vi "一体站流程自动启动.vi"(11 "参数":T1={"CODCr"={"启动测量模式"={"测量模式"=enum."水样测量"}, "确定按钮"=TRUE}, "参数启用"={"多参数"=FALSE, "CODMn"=FALSE, "总磷总氮"=FALSE, "氨氮"=FALSE, "CODcr"=FALSE}}) -> ()   [LabVIEW 2016, in "PLC.lvlib"]
uses:
  PLC.lvlib
  API/CodCr/CodCr.lvlib
panel:
  out "枚举":enum16{"初始化", "采配水启动", "等待", "配水", "排水", "结束"}(ring)
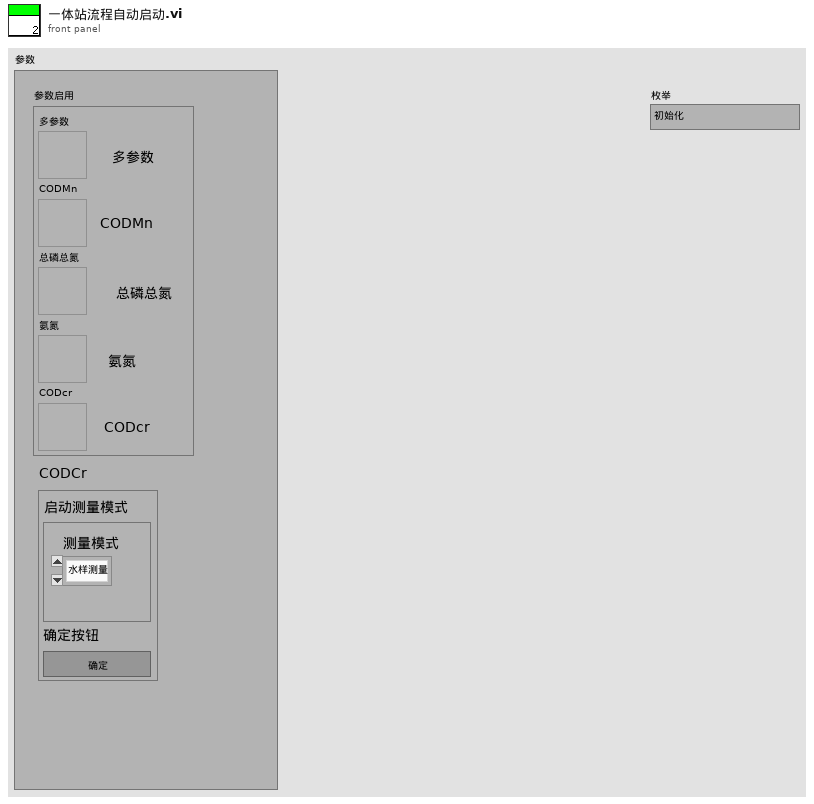
[diagram p1: front panel]
types:
  T1 = cluster{"CODCr":cluster{"启动测量模式":cluster{"测量模式":enum16{"水样测量", "标样核查", "零点核查", "跨度核查", "空白测试", "加标回收", "平行样", "校零", "校标"}}, "确定按钮":bool}, "参数启用":cluster{"多参数":bool, "CODMn":bool, "总磷总氮":bool, "氨氮":bool, "CODcr":bool}}
  T2 = cluster{"命令":string, cluster{"starting address":u16, "holding register value":u16}}
  T3 = cluster{"测量模式":enum16{"水样测量", "标样核查", "零点核查", "跨度核查", "空白测试", "加标回收", "平行样", "校零", "校标"}}
  T4 = cluster{"时间标识":timestamp, "设备":string, "日志信息":string, "流程参数":string}
  T5 = cluster{"时间标识":timestamp, "设备":string, "日志信息":string}
  T6 = enum16{"空闲", "水样测试", "标样核查", "零点核查", "跨度核查", "空白测试", "平行样测试", "加标回收", "空白校准", "标样校准", "初始化（清洗）"}
  T7 = enum16{"待机", "启动氨氮", "氨氮测量中", "启动总磷", "总磷测量中", "结束"}
  T8 = cluster{"站号":u16, "量程切换":enum32{"H", "L", "AUTO"}, "控制命令":enum16{"启动测量", "标样核查", "零点核查", "跨度核查", "空白测试", "平行样测试", "加标回收", "空白校准", "标样校准", "初始化（清洗）", "停止测试", "仪器重启", "校时", "模式设置", "测量间隔设置"}, "模式设置":enum16{"待机", "连续模式", "周期模式", "定点模式", "受控模式", "手动模式"}, "测量间隔":u16}
  T9 = cluster{"测量模式":enum16{"待机", "水样测试", "标样核查", "零点核查", "跨度核查", "空白测试", "平行样测试", "加标回收", "空白校准", "标样校准", "初始化（清洗）"}, "数据标记表":string, "测量时间":dbl}
  T10 = enum16{"待机", "水样测试", "标样核查", "零点核查", "跨度核查", "空白测试", "平行样测试", "加标回收", "空白校准", "标样校准", "初始化（清洗）"}
  T11 = cluster{"R0":i16, "R1":i16, "R2":i16, "R3":i16, "R4":i16, "R5":i16, "R6":i16, "R7":i16, "R8":i16, "R9":i16, "R10":i16, "R11":i16, "R12":i16, "R13":i16, "R14":i16, "R15":i16, "R16":i16, "R17":i16, "R18":i16, "R19":i16, "R20":i16, "R21":i16, "R22":i16, "R23":i16, "R24":i16, "R25":i16, "R26":i16, "R27":i16, "R28":i16, "R29":i16, "R30":i16, "R31":i16, "R32":i16, "R33":i16, "R34":i16, "R35":i16, "R36":i16, "R37":i16, "R38":i16, "R39":i16, "R40":i16, "R41":i16, "R42":i16, "R43":i16, "R44":i16, "R45":i16, "R46":i16, "R47":i16, "R48":i16, "R49":i16, "R50":i16, "R51":i16, "R52":i16, "R53":i16, "R54":i16, "R55":i16}
  T12 = cluster{"系统时间":timestamp, "工作状态":enum16{"空闲", "水样测试", "标样核查", "零点核查", "跨度核查", "空白测试", "平行样测试", "加标回收", "空白校准", "标样校准", "初始化（清洗）"}, "测量模式":enum16{"待机", "连续模式", "周期模式", "定点模式", "受控模式", "手动模式"}, "告警代码":enum16{"无告警", "缺试剂告警", "缺水样告警", "缺蒸馏水告警", "缺标液告警", "仪表漏液告警", "标定异常告警", "超量程告警", "加热异常", "低试剂预警", "超上限告警", "超下限告警", "仪表内部其他异常", "滴定异常告警", "电极异常告警", "量程切换告警", "参数设置告警", "PH电极电位异常", "电导率电极异常", "浊度光度异常", "溶解氧电极异常", "溶解氧光强异常", "温度异常告警", "PH异常告警", "溶解氧异常告警", "电导率异常告警", "浊度异常告警", "叶绿素异常告警", "藻密度异常告警", "蓝绿藻异常告警", "ORP异常告警", "氨氮异常告警", "清洁刷异常告警", "SD卡异常告警", "蓝牙异常告警", "Wifi异常告警", "流程异常告警"}, "故障代码":enum16{"无故障", "电机故障", "温度故障", "通讯故障", "滴定故障"}, "日志代码":u16, "软件版本":u16, "F0":sgl, "F1":sgl, "F2":sgl, "F3":sgl, "T":sgl, "H":sgl, "id":u16, "flowid":u16, "量程":u16, "总磷控温温度1":sgl, "营养盐控温温度2":sgl, "ADC":sgl}
  T13 = cluster{"因子编码":u32, "单位":u16, "标样参考值":sgl, "水样数据时间":timestamp, "水样实测值":sgl, "水样数据标识":string, "标样数据时间":timestamp, "标样实测值":sgl, "标样数据标识":string, "空白数据时间":timestamp, "空白实测值":sgl, "空白数据标识":string, "零点核查数据时间":timestamp, "零点核查实测值":sgl, "零点核查数据标识":string, "跨度核查数据时间":timestamp, "跨度核查实测值":sgl, "跨度核查数据标识":string, "加标回收数据时间":timestamp, "加标回收实测值":sgl, "加标回收数据标识":string, "平行样数据时间":timestamp, "平行样实测值":sgl, "平行样数据标识":string, "F0":sgl, "F1":sgl, "F2":sgl, "F3":sgl, "F4":sgl, "F5":sgl, "F6":sgl, "F7":sgl, "温度":sgl, "湿度":sgl, "X值":sgl}
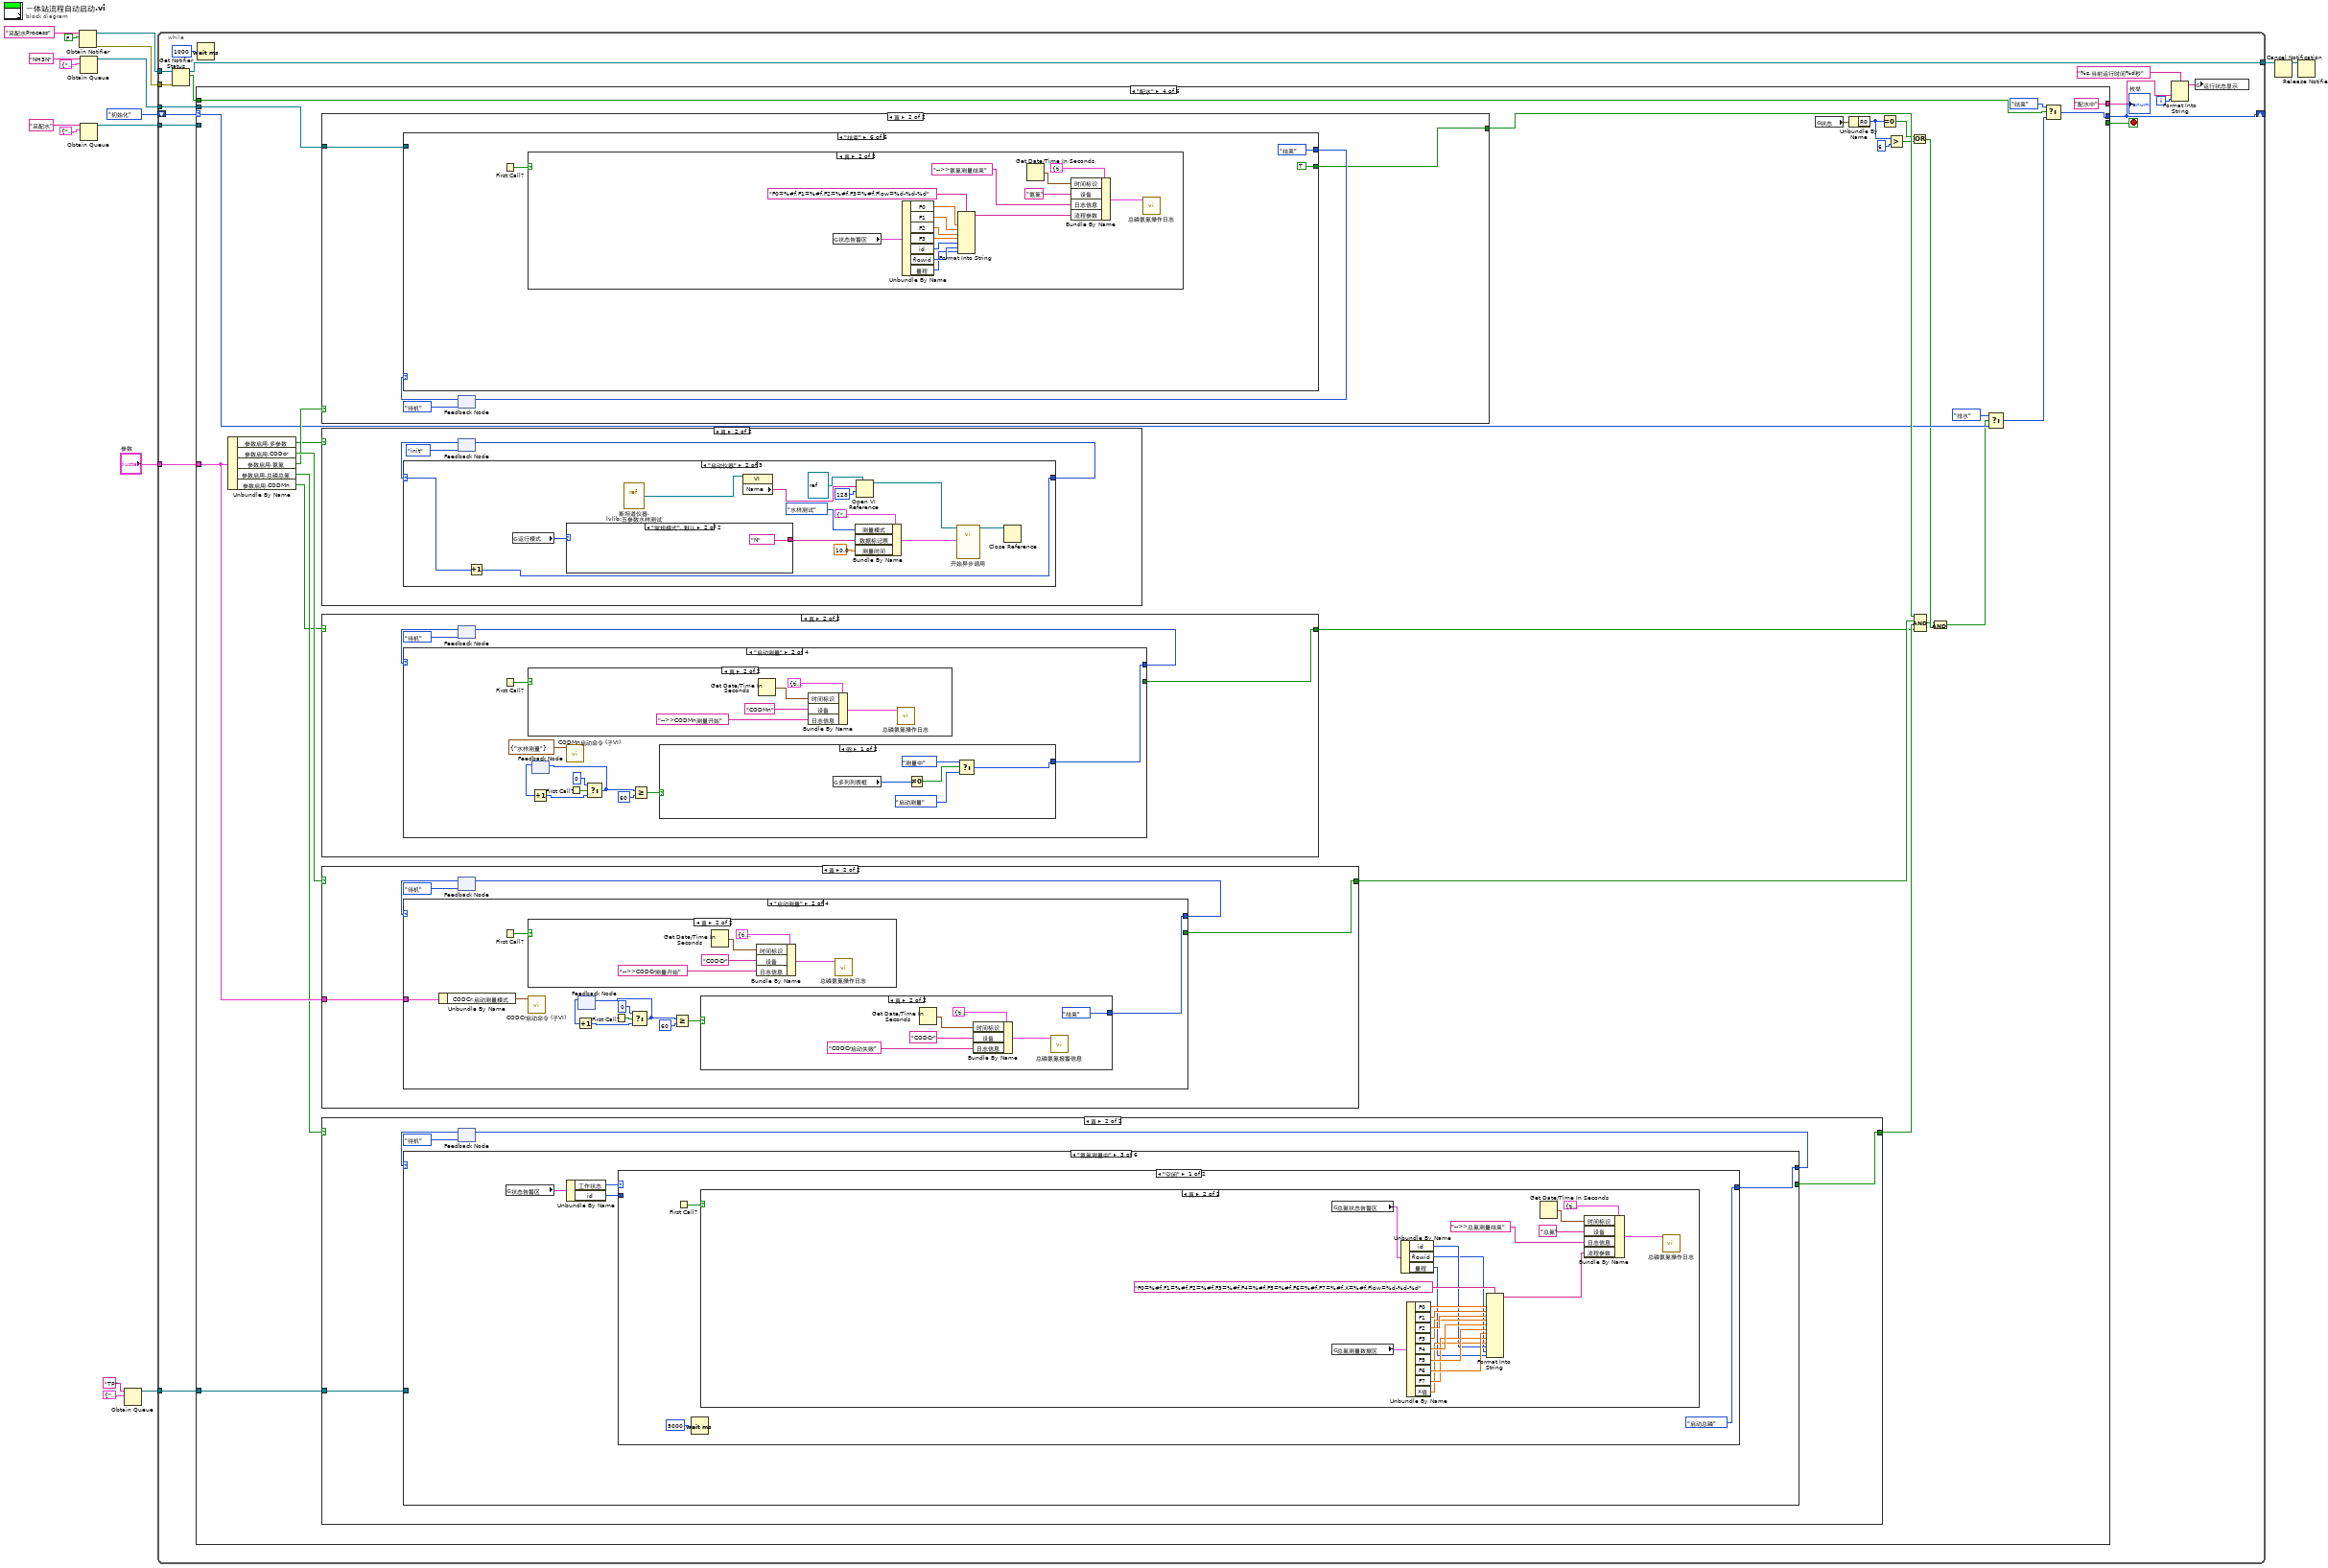
[diagram p0: block diagram]
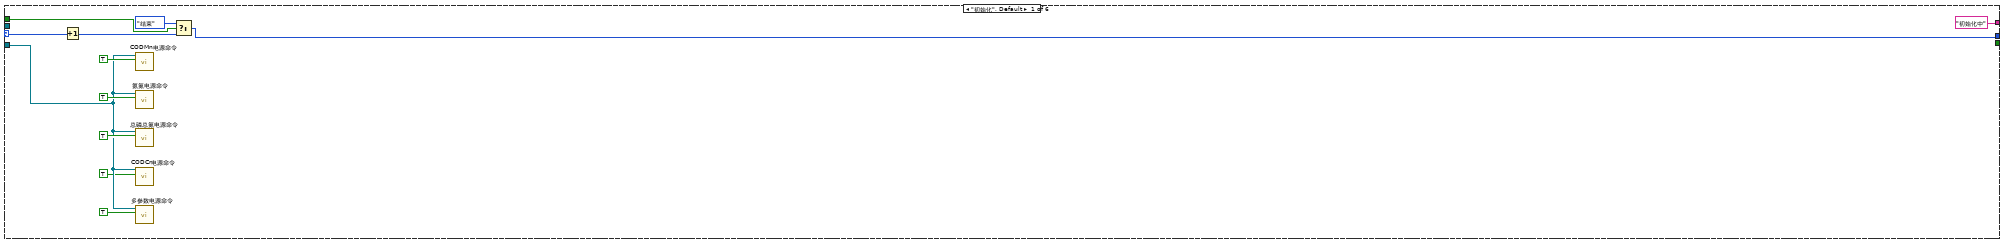
[diagram p2: hidden frame]
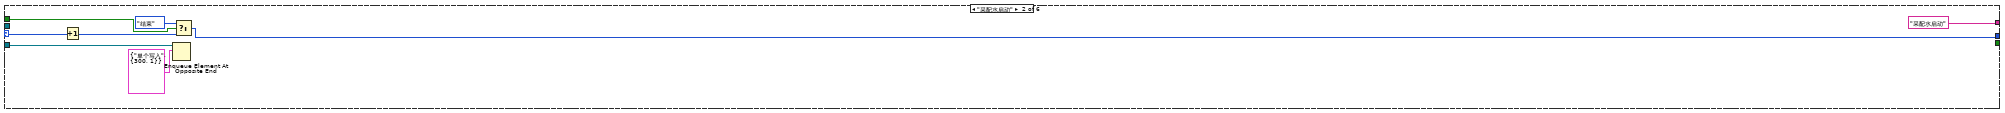
[diagram p3: hidden frame]
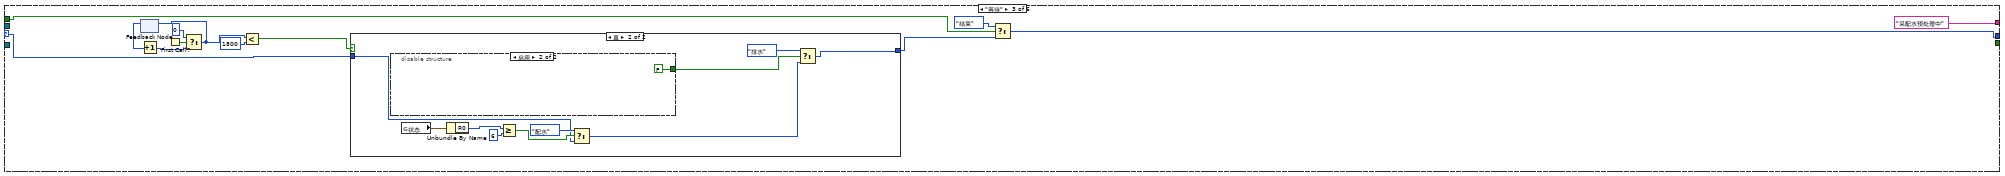
[diagram p4: hidden frame]
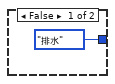
[diagram p5: hidden frame]
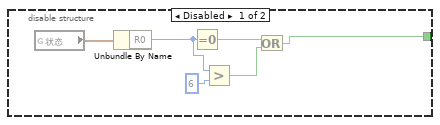
[diagram p6: hidden frame]
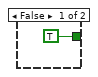
[diagram p7: hidden frame]
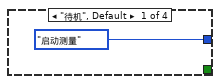
[diagram p8: hidden frame]
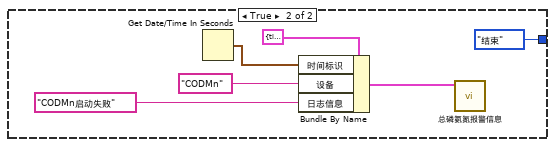
[diagram p10: hidden frame]
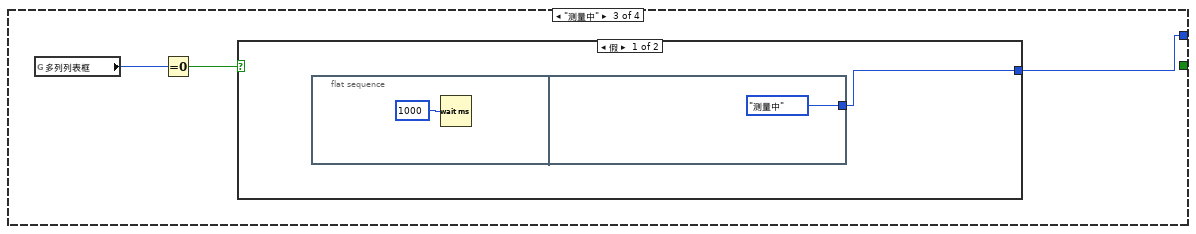
[diagram p11: hidden frame]
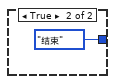
[diagram p12: hidden frame]
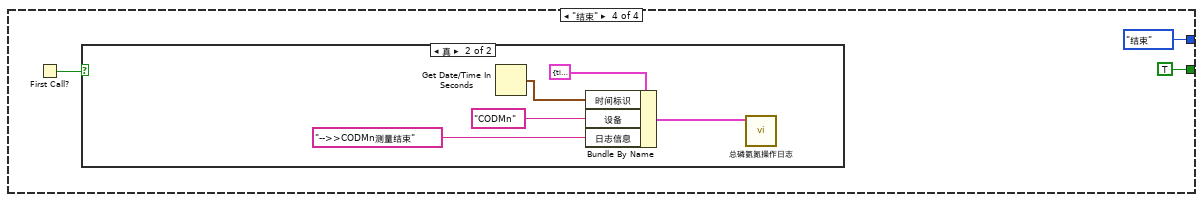
[diagram p13: hidden frame]
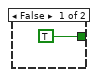
[diagram p15: hidden frame]
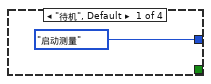
[diagram p16: hidden frame]
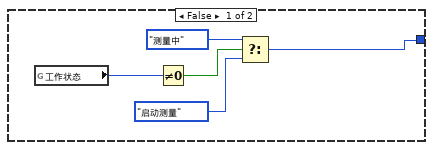
[diagram p18: hidden frame]
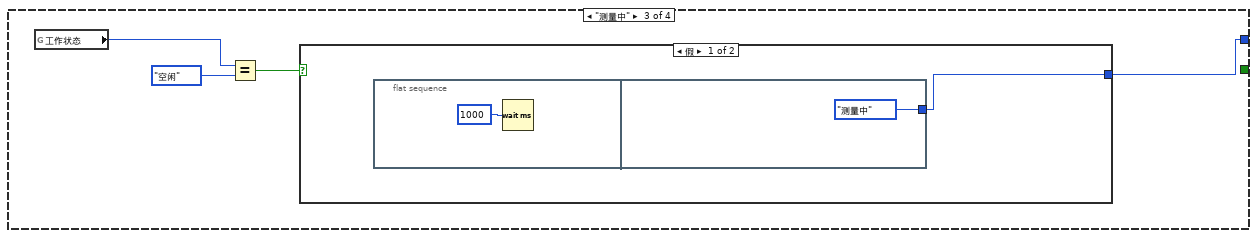
[diagram p19: hidden frame]
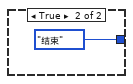
[diagram p20: hidden frame]
diagram:
  n1 = Obtain Notifier(name (unnamed)="采配水Process" ("名称（未命名）"), notification data type=FALSE) -> (notifier out=w2:refnum<notifier>, error out=w1:errorcluster)  [unwired: 2 in, 1 out]
  n2 = Obtain Queue(name (unnamed)="NH3N" ("名称（未命名）"), element data type=cluster{"命令":string, "data":variant} {"命令"="", "data"=variant}) -> (queue out=w4:refnum<queue>)  [unwired: 3 in, 2 out]
  n3 = Obtain Queue(name (unnamed)="采配水" ("名称（未命名）"), element data type=cluster{"命令":string, "数据":variant} {"命令"="", "数据"=variant}) -> (queue out=w15:refnum<queue>)  [unwired: 3 in, 2 out]
  n4 = Obtain Queue(name (unnamed)="TP" ("名称（未命名）"), element data type=cluster{"命令":string, "data":variant} {"命令"="", "data"=variant}) -> (queue out=w3:refnum<queue>)  [unwired: 3 in, 2 out]
  n5 = while {
    tunnel: w15 -> [w33]
    shift-right: [w31] -> _
    shift-left: enum16{"初始化", "采配水启动", "等待", "配水", "排水", "结束"}."初始化" ("枚举") -> [w32]
    tunnel: w4 -> [w29]
    tunnel: "参数" -> [w28]
    tunnel: w2 -> [w27]
    tunnel: [w26] -> w8
    tunnel: w3 -> [w21]
    tunnel: w1 -> [w18]
    i -> [w23]
    stop <- w19 stop-if-true
    n6 = Get Notifier Status(notifier=w27, error in (no error)=w18) -> (notifier out=w26:refnum<notifier>, current notification=w22:bool)  [unwired: 3 out]
    n7 = case shown="\"配水\"" w32 {
      selector: w32 -> [w45 w51 w64 w89 w497 w505]
      tunnel: w33 -> [w35 w52 _ _ w498 w501]
      tunnel: [w41 w46 w54 w108 w492 w504] -> w31
      tunnel: [_ _ _ _ _ TRUE] -> w19
      tunnel: w29 -> [_ _ _ w106 _ _]
      tunnel: w28 -> [_ _ _ w103 _ _]
      tunnel: ["初始化中" ("输入 1") "采配水启动" ("输入 1") "采配水预处理中" ("输入 1") "配水中" ("输入 1") "排水中" ("输入 1") "结束" ("输入 1")] -> w24
      tunnel: w22 -> [w43 w48 w56 w109 w494 w500]
      tunnel: w21 -> [_ _ _ w107 _ _]
      frame "初始化", Default {
        n8 = Increment(x=w45) -> (x+1=w42:enum16{"初始化", "采配水启动", "等待", "配水", "排水", "结束"})
        n9 = call "CODMn电源命令.vi"("通电/断电"=TRUE, "队列"=w35) -> ()  [unwired: 9 in, 1 out]
        n10 = call "氨氮电源命令.vi"("通电/断电"=TRUE, "队列"=w35) -> ()  [unwired: 9 in, 1 out]
        n11 = call "总磷总氮电源命令.vi"("通电/断电"=TRUE, "队列"=w35) -> ()  [unwired: 9 in, 1 out]
        n12 = call "CODCr电源命令.vi"("通电/断电"=TRUE, "队列"=w35) -> ()  [unwired: 9 in, 1 out]
        n13 = call "多参数电源命令.vi"("通电/断电"=TRUE, "队列"=w35) -> ()  [unwired: 9 in, 1 out]
        n14 = Select(t=enum16{"初始化", "采配水启动", "等待", "配水", "排水", "结束"}."结束", s=w43, f=w42) -> (s? t:f=w41:enum16{"初始化", "采配水启动", "等待", "配水", "排水", "结束"})
      }
      frame "采配水启动" {
        n15 = Increment(x=w51) -> (x+1=w47:enum16{"初始化", "采配水启动", "等待", "配水", "排水", "结束"})
        n16 = Enqueue Element At Opposite End(queue=w52, element=T2 {"命令"="单个写入", {"starting address"=300, "holding register value"=1}} ("元素")) -> ()  [unwired: 2 in, 3 out]
        n17 = Select(t=enum16{"初始化", "采配水启动", "等待", "配水", "排水", "结束"}."结束", s=w48, f=w47) -> (s? t:f=w46:enum16{"初始化", "采配水启动", "等待", "配水", "排水", "结束"})
      }
      frame "等待" {
        n18 = feedback #1() -> (w61:i32)  [unwired: 1 in]
        n19 = Increment(x=w61) -> (x+1=w60:i32)
        n20 = First Call?() -> (First Call?: T/F=w62:bool)
        n21 = Select(t=0, s=w62, f=w60) -> (s? t:f=w59:i32)
        n22 = feedback-in #1(w59) -> ()
        n23 = Less?(x=w59, y=1800) -> (x < y?=w65:bool)
        n24 = case shown="真" w65 {
          tunnel: w64 -> [_ w70]
          tunnel: [enum16{"初始化", "采配水启动", "等待", "配水", "排水", "结束"}."排水" ("枚举") w68] -> w55
          frame False {
          }
          frame True {
            n25 = disable-structure shown="启用" {
              disable-tunnel: [w83 FALSE] -> w72
              frame Disabled {
                n26 = global read "采配水全局变量.vi" "状态"() -> (w78:T11)
                n27 = Unbundle By Name(w78) -> ("R0"=w79:i16)
                n28 = Equal To 0?(x=w79) -> (x = 0?=w82:bool)
                n29 = Greater?(x=w79, y=i16 6) -> (0:w81:bool)
                n30 = Or(x=w82, y=w81) -> (x .or. y?=w83:bool)
              }
              frame Enabled {
              }
            }
            n31 = global read "采配水全局变量.vi" "状态"() -> (w77:T11)
            n32 = Unbundle By Name(w77) -> ("R0"=w76:i16)
            n33 = Greater Or Equal?(x=w76, y=i16 6) -> (x >= y?=w74:bool)
            n34 = Select(t=enum16{"初始化", "采配水启动", "等待", "配水", "排水", "结束"}."配水" ("枚举"), s=w74, f=w70) -> (s? t:f=w69:enum16{"初始化", "采配水启动", "等待", "配水", "排水", "结束"})
            n35 = Select(t=enum16{"初始化", "采配水启动", "等待", "配水", "排水", "结束"}."排水" ("枚举"), s=w72, f=w69) -> (s? t:f=w68:enum16{"初始化", "采配水启动", "等待", "配水", "排水", "结束"})
          }
        }
        n36 = Select(t=enum16{"初始化", "采配水启动", "等待", "配水", "排水", "结束"}."结束", s=w56, f=w55) -> (s? t:f=w54:enum16{"初始化", "采配水启动", "等待", "配水", "排水", "结束"})
      }
      frame "配水" {
        n37 = Unbundle By Name(w103) -> ("参数启用.多参数"=w96:bool, "参数启用.CODcr"=w100:bool, "参数启用.氨氮"=w99:bool, "参数启用.总磷总氮"=w98:bool, "参数启用.CODMn"=w97:bool)
        n38 = case shown="真" w99 {
          tunnel: [TRUE w367] -> w105
          tunnel: w106 -> [_ w366]
          frame False {
          }
          frame True {
            n39 = feedback #2(T7."待机") -> (w369:T7)
            n40 = case shown="\"结束\"" w369 {
              tunnel: [T7."启动氨氮" w383 w412 w430 w444 T7."结束"] -> w368
              tunnel: [_ _ _ _ _ TRUE] -> w367
              tunnel: w366 -> [_ w374 _ w421 _ _]
              frame "待机", Default {
              }
              frame "启动氨氮" {
                n41 = First Call?() -> (First Call?: T/F=w372:bool)
                n42 = case shown="真" w372 {
                  frame False {
                  }
                  frame True {
                    n43 = global read "VAR总磷氨氮全局变量.vi" "状态告警区"() -> (w393:T12)
                    n44 = Unbundle By Name(w393) -> ("F0"=w391:sgl, "F1"=w390:sgl, "F2"=w389:sgl, "F3"=w388:sgl, "id"=w387:u16, "flowid"=w386:u16, "量程"=w385:u16)
                    n45 = Format Into String(format string="F0=%#f,F1=%#f,F2=%#f,F3=%#f,%d-%d-%d" ("格式字符串"), w391, w390, w389, w388, w387, w386, w385) -> (resulting string=w384:string)  [unwired: 2 in, 1 out]
                    n46 = Get Date/Time In Seconds() -> (seconds since 1Jan1904=w396:timestamp)
                    n47 = Bundle By Name(cluster=T4 {"时间标识"=timestamp(0 s since 1904-01-01), "设备"="", "日志信息"="", "流程参数"=""} ("data in"), "时间标识"=w396, "设备"="氨氮", "日志信息"="-->>氨氮测量开始" ("设备"), "流程参数"=w384) -> (w397:T4)
                    n48 = call "总磷氨氮操作日志.vi"("data in"=w397) -> ()  [unwired: 11 in]
                  }
                }
                n49 = call "总磷氨氮启动命令.vi"("参数"=T8 {"站号"=3, "量程切换"=enum."AUTO", "控制命令"=enum."启动测量", "模式设置"=enum."待机", "测量间隔"=0}) -> ("启动命令"=w375:cluster{"命令":string, "data":variant})  [unwired: 10 in]
                n50 = Enqueue Element(queue=w374, element=w375) -> ()  [unwired: 2 in, 3 out]
                n51 = feedback #3() -> (w380:i32)  [unwired: 1 in]
                n52 = Increment(x=w380) -> (x+1=w379:i32)
                n53 = First Call?() -> (First Call?: T/F=w381:bool)
                n54 = Select(t=0, s=w381, f=w379) -> (s? t:f=w378:i32)
                n55 = feedback-in #3(w378) -> ()
                n56 = Greater Or Equal?(x=w378, y=60) -> (x >= y?=w376:bool)
                n57 = case shown="真" w376 {
                  tunnel: [w402 T7."结束"] -> w383
                  frame False {
                    n58 = global read "VAR总磷氨氮全局变量.vi" "状态告警区"() -> (w399:T12)
                    n59 = Unbundle By Name(w399) -> ("工作状态"=w404:T6)
                    n60 = Not Equal To 0?(x=w404) -> (x != 0?=w403:bool)
                    n61 = Select(t=T7."氨氮测量中", s=w403, f=T7."启动氨氮") -> (s? t:f=w402:T7)
                  }
                  frame True {
                    n62 = Get Date/Time In Seconds() -> (seconds since 1Jan1904=w409:timestamp)
                    n63 = Bundle By Name(cluster=T5 {"时间标识"=timestamp(0 s since 1904-01-01), "设备"="", "日志信息"=""} ("data in"), "时间标识"=w409, "设备"="氨氮", "日志信息"="氨氮启动失败") -> (w405:T5)
                    n64 = call "总磷氨氮报警信息.vi"("data in"=w405) -> ()  [unwired: 11 in]
                  }
                }
              }
              frame "氨氮测量中" {
                n65 = global read "VAR总磷氨氮全局变量.vi" "状态告警区"() -> (w411:T12)
                n66 = Unbundle By Name(w411) -> ("工作状态"=w414:T6, "id"=w413:u16)
                n67 = case shown="\"水样测试\", 默认" w414 {
                  tunnel: [T7."结束" w416] -> w412
                  tunnel: w413 -> [_ w417]
                  frame "空闲" {
                  }
                  frame "水样测试", Default {
                    n68 = case shown="76, 默认" w417 {
                      tunnel: [T7."氨氮测量中" T7."总磷测量中"] -> w416
                      frame 76, Default {
                      }
                      frame 131 {
                      }
                    }
                  }
                }
              }
              frame "启动总磷" {
                n69 = call "总磷氨氮启动命令.vi"("参数"=T8 {"站号"=1, "量程切换"=enum."AUTO", "控制命令"=enum."启动测量", "模式设置"=enum."待机", "测量间隔"=0}) -> ("启动命令"=w422:cluster{"命令":string, "data":variant})  [unwired: 10 in]
                n70 = Enqueue Element(queue=w421, element=w422) -> ()  [unwired: 2 in, 3 out]
                n71 = feedback #4() -> (w427:i32)  [unwired: 1 in]
                n72 = Increment(x=w427) -> (x+1=w426:i32)
                n73 = First Call?() -> (First Call?: T/F=w428:bool)
                n74 = Select(t=0, s=w428, f=w426) -> (s? t:f=w425:i32)
                n75 = feedback-in #4(w425) -> ()
                n76 = Greater Or Equal?(x=w425, y=60) -> (x >= y?=w423:bool)
                n77 = case shown="假" w423 {
                  tunnel: [w434 T7."结束"] -> w430
                  frame False {
                    n78 = global read "VAR总磷氨氮全局变量.vi" "状态告警区"() -> (w431:T12)
                    n79 = Unbundle By Name(w431) -> ("工作状态"=w435:T6)
                    n80 = Not Equal To 0?(x=w435) -> (x != 0?=w436:bool)
                    n81 = Select(t=T7."总磷测量中", s=w436, f=T7."启动总磷") -> (s? t:f=w434:T7)
                  }
                  frame True {
                    n82 = Get Date/Time In Seconds() -> (seconds since 1Jan1904=w442:timestamp)
                    n83 = Bundle By Name(cluster=T5 {"时间标识"=timestamp(0 s since 1904-01-01), "设备"="", "日志信息"=""} ("data in"), "时间标识"=w442, "设备"="总磷", "日志信息"="总磷启动失败") -> (w437:T5)
                    n84 = call "总磷氨氮报警信息.vi"("data in"=w437) -> ()  [unwired: 11 in]
                  }
                }
              }
              frame "总磷测量中" {
                n85 = global read "VAR总磷氨氮全局变量.vi" "状态告警区"() -> (w443:T12)
                n86 = Unbundle By Name(w443) -> ("工作状态"=w446:T6, "id"=w445:u16)
                n87 = case shown="\"水样测试\", 默认" w446 {
                  tunnel: [T7."结束" w448] -> w444
                  tunnel: w445 -> [_ w449]
                  frame "空闲" {
                  }
                  frame "水样测试", Default {
                    n88 = case shown="76, 默认" w449 {
                      tunnel: [T7."氨氮测量中" T7."总磷测量中"] -> w448
                      frame 76, Default {
                      }
                      frame 131 {
                      }
                    }
                  }
                }
              }
              frame "结束" {
                n89 = First Call?() -> (First Call?: T/F=w452:bool)
                n90 = case shown="真" w452 {
                  frame False {
                  }
                  frame True {
                    n91 = global read "VAR总磷氨氮全局变量.vi" "状态告警区"() -> (w464:T12)
                    n92 = Unbundle By Name(w464) -> ("F0"=w462:sgl, "F1"=w461:sgl, "F2"=w460:sgl, "F3"=w459:sgl, "id"=w458:u16, "flowid"=w457:u16, "量程"=w456:u16)
                    n93 = Format Into String(format string="F0=%#f,F1=%#f,F2=%#f,F3=%#f,Flow=%d-%d-%d" ("格式字符串"), w462, w461, w460, w459, w458, w457, w456) -> (resulting string=w455:string)  [unwired: 2 in, 1 out]
                    n94 = Get Date/Time In Seconds() -> (seconds since 1Jan1904=w467:timestamp)
                    n95 = Bundle By Name(cluster=T4 {"时间标识"=timestamp(0 s since 1904-01-01), "设备"="", "日志信息"="", "流程参数"=""} ("data in"), "时间标识"=w467, "设备"="氨氮", "日志信息"="-->>氨氮测量结束" ("设备"), "流程参数"=w455) -> (w468:T4)
                    n96 = call "总磷氨氮操作日志.vi"("data in"=w468) -> ()  [unwired: 11 in]
                  }
                }
              }
            }
            n97 = feedback-in #2(w368) -> ()
          }
        }
        n98 = case shown="真" w96 {
          frame False {
          }
          frame True {
            n99 = feedback #5(enum16{"init", "启动仪器", "测量中"}."init") -> (w471:enum16{"init", "启动仪器", "测量中"})
            n100 = case shown="\"启动仪器\"" w471 {
              selector: w471 -> [w474 w488 _]
              tunnel: [w473 w487 enum16{"init", "启动仪器", "测量中"}."测量中"] -> w472
              frame "init", Default {
                n101 = Increment(x=w474) -> (x+1=w473:enum16{"init", "启动仪器", "测量中"})
              }
              frame "启动仪器" {
                n102 = Increment(x=w488) -> (x+1=w487:enum16{"init", "启动仪器", "测量中"})
                n103 = global read "系统变量.vi" "运行模式"() -> (w476:enum16{"维护模式", "常规模式", "应急模式", "质控模式"})
                n104 = case shown="\"常规模式\", 默认" w476 {
                  tunnel: ["M" ("数据标记表") "N" ("数据标记表")] -> w475
                  frame "维护模式" {
                  }
                  frame "常规模式", Default {
                  }
                }
                n105 = vi-ref "斯坦道仪器.lvlib:五参数水样测试.vi"() -> (w486:refnum<vi>)
                n106 = property class="VI"(reference=w486) -> ("Name"=w485:string)  [unwired: 1 in, 2 out]
                n107 = Bundle By Name(cluster=T9 {"测量模式"=enum."待机", "数据标记表"="", "测量时间"=0.0} ("启动参数"), "测量模式"=T10."水样测试", "数据标记表"=w475, "测量时间"=10.0) -> (w477:T9)
                n108 = Open VI Reference(type specifier VI Refnum (for type only)=refnum<vi> refnum ("类型说明符VI引用句柄（仅用于类型）"), vi path=w485, options=128 ("选项")) -> (vi reference=w480:refnum<vi>)  [unwired: 3 in, 1 out]
                n109 = call-by-ref "开始异步调用"(reference=w480, "启动参数"=w477) -> (reference out=w479:refnum<vi>)  [unwired: 12 in, 1 out]
                n110 = Close Reference(reference=w479) -> ()  [unwired: 1 in, 1 out]
              }
              frame "测量中" {
              }
            }
            n111 = feedback-in #5(w472) -> ()
          }
        }
        n112 = case shown="真" w97 {
          tunnel: [TRUE w113] -> w101
          frame False {
          }
          frame True {
            n113 = feedback #6(enum16{"待机", "启动测量", "测量中", "结束"}."待机") -> (w115:enum16{"待机", "启动测量", "测量中", "结束"})
            n114 = case shown="\"启动测量\"" w115 {
              tunnel: [enum16{"待机", "启动测量", "测量中", "结束"}."启动测量" w127 w146 enum16{"待机", "启动测量", "测量中", "结束"}."结束"] -> w114
              tunnel: [_ _ _ TRUE] -> w113
              frame "待机", Default {
              }
              frame "启动测量" {
                n115 = First Call?() -> (First Call?: T/F=w118:bool)
                n116 = case shown="真" w118 {
                  frame False {
                  }
                  frame True {
                    n117 = Get Date/Time In Seconds() -> (seconds since 1Jan1904=w132:timestamp)
                    n118 = Bundle By Name(cluster=T4 {"时间标识"=timestamp(0 s since 1904-01-01), "设备"="", "日志信息"="", "流程参数"=""} ("data in"), "时间标识"=w132, "设备"="CODMn", "日志信息"="-->>CODMn测量开始") -> (w128:T4)
                    n119 = call "总磷氨氮操作日志.vi"("data in"=w128) -> ()  [unwired: 11 in]
                  }
                }
                n120 = feedback #7() -> (w123:i32)  [unwired: 1 in]
                n121 = Increment(x=w123) -> (x+1=w124:i32)
                n122 = call "CODMn启动命令 (子VI).vi"("启动测量模式"=T3 {"测量模式"=enum."水样测量"}) -> ()  [unwired: 11 in]
                n123 = First Call?() -> (First Call?: T/F=w122:bool)
                n124 = Select(t=0, s=w122, f=w124) -> (s? t:f=w125:i32)
                n125 = feedback-in #7(w125) -> ()
                n126 = Greater Or Equal?(x=w125, y=60) -> (x >= y?=w120:bool)
                n127 = case shown="假" w120 {
                  tunnel: [w134 enum16{"待机", "启动测量", "测量中", "结束"}."结束"] -> w127
                  frame False {
                    n128 = global read "运行时序全局变量.vi" "多列列表框"() -> (w133:i32)
                    n129 = Not Equal To 0?(x=w133) -> (x != 0?=w135:bool)
                    n130 = Select(t=enum16{"待机", "启动测量", "测量中", "结束"}."测量中", s=w135, f=enum16{"待机", "启动测量", "测量中", "结束"}."启动测量") -> (s? t:f=w134:enum16{"待机", "启动测量", "测量中", "结束"})
                  }
                  frame True {
                    n131 = Get Date/Time In Seconds() -> (seconds since 1Jan1904=w138:timestamp)
                    n132 = Bundle By Name(cluster=T5 {"时间标识"=timestamp(0 s since 1904-01-01), "设备"="", "日志信息"=""} ("data in"), "时间标识"=w138, "设备"="CODMn", "日志信息"="CODMn启动失败") -> (w142:T5)
                    n133 = call "总磷氨氮报警信息.vi"("data in"=w142) -> ()  [unwired: 11 in]
                  }
                }
              }
              frame "测量中" {
                n134 = global read "运行时序全局变量.vi" "多列列表框"() -> (w145:i32)
                n135 = Equal To 0?(x=w145) -> (x = 0?=w144:bool)
                n136 = case shown="假" w144 {
                  tunnel: [w147 enum16{"待机", "启动测量", "测量中", "结束"}."结束"] -> w146
                  frame False {
                    n137 = flat-sequence {
                      tunnel: [enum16{"待机", "启动测量", "测量中", "结束"}."测量中"] -> w147
                      frame #0 {
                        n138 = Wait (ms)(milliseconds to wait=u32 1000 ("等待时间（毫秒）")) -> ()  [unwired: 1 out]
                      }
                      frame #1 {
                      }
                    }
                  }
                  frame True {
                  }
                }
              }
              frame "结束" {
                n139 = First Call?() -> (First Call?: T/F=w151:bool)
                n140 = case shown="真" w151 {
                  frame False {
                  }
                  frame True {
                    n141 = Get Date/Time In Seconds() -> (seconds since 1Jan1904=w158:timestamp)
                    n142 = Bundle By Name(cluster=T4 {"时间标识"=timestamp(0 s since 1904-01-01), "设备"="", "日志信息"="", "流程参数"=""} ("data in"), "时间标识"=w158, "设备"="CODMn", "日志信息"="-->>CODMn测量结束") -> (w154:T4)
                    n143 = call "总磷氨氮操作日志.vi"("data in"=w154) -> ()  [unwired: 11 in]
                  }
                }
              }
            }
            n144 = feedback-in #6(w114) -> ()
          }
        }
        n145 = case shown="真" w100 {
          tunnel: [TRUE w161] -> w102
          tunnel: w103 -> [_ w160]
          frame False {
          }
          frame True {
            n146 = feedback #8(enum16{"待机", "启动测量", "测量中", "结束"}."待机") -> (w163:enum16{"待机", "启动测量", "测量中", "结束"})
            n147 = case shown="\"启动测量\"" w163 {
              tunnel: [enum16{"待机", "启动测量", "测量中", "结束"}."启动测量" w175 w196 enum16{"待机", "启动测量", "测量中", "结束"}."结束"] -> w162
              tunnel: w160 -> [_ w176 _ _]
              tunnel: [_ _ _ TRUE] -> w161
              frame "待机", Default {
              }
              frame "启动测量" {
                n148 = Unbundle By Name(w176) -> ("CODCr.启动测量模式"=w174:T3)
                n149 = First Call?() -> (First Call?: T/F=w166:bool)
                n150 = case shown="真" w166 {
                  frame False {
                  }
                  frame True {
                    n151 = Get Date/Time In Seconds() -> (seconds since 1Jan1904=w181:timestamp)
                    n152 = Bundle By Name(cluster=T4 {"时间标识"=timestamp(0 s since 1904-01-01), "设备"="", "日志信息"="", "流程参数"=""} ("data in"), "时间标识"=w181, "设备"="CODCr", "日志信息"="-->>CODCr测量开始") -> (w177:T4)
                    n153 = call "总磷氨氮操作日志.vi"("data in"=w177) -> ()  [unwired: 11 in]
                  }
                }
                n154 = call "CODCr启动命令 (子VI).vi"("启动测量模式"=w174) -> ()  [unwired: 11 in]
                n155 = feedback #9() -> (w170:i32)  [unwired: 1 in]
                n156 = Increment(x=w170) -> (x+1=w171:i32)
                n157 = First Call?() -> (First Call?: T/F=w169:bool)
                n158 = Select(t=0, s=w169, f=w171) -> (s? t:f=w172:i32)
                n159 = feedback-in #9(w172) -> ()
                n160 = Greater Or Equal?(x=w172, y=60) -> (x >= y?=w167:bool)
                n161 = case shown="真" w167 {
                  tunnel: [w182 enum16{"待机", "启动测量", "测量中", "结束"}."结束"] -> w175
                  frame False {
                    n162 = global read "CODCr工作状态.vi" "工作状态"() -> (w183:T6)
                    n163 = Not Equal To 0?(x=w183) -> (x != 0?=w184:bool)
                    n164 = Select(t=enum16{"待机", "启动测量", "测量中", "结束"}."测量中", s=w184, f=enum16{"待机", "启动测量", "测量中", "结束"}."启动测量") -> (s? t:f=w182:enum16{"待机", "启动测量", "测量中", "结束"})
                  }
                  frame True {
                    n165 = Get Date/Time In Seconds() -> (seconds since 1Jan1904=w187:timestamp)
                    n166 = Bundle By Name(cluster=T5 {"时间标识"=timestamp(0 s since 1904-01-01), "设备"="", "日志信息"=""} ("data in"), "时间标识"=w187, "设备"="CODCr", "日志信息"="CODCr启动失败") -> (w191:T5)
                    n167 = call "总磷氨氮报警信息.vi"("data in"=w191) -> ()  [unwired: 11 in]
                  }
                }
              }
              frame "测量中" {
                n168 = global read "CODCr工作状态.vi" "工作状态"() -> (w195:T6)
                n169 = Equal?(x=w195, y=T6."空闲" ("工作状态")) -> (x = y?=w194:bool)
                n170 = case shown="假" w194 {
                  tunnel: [w197 enum16{"待机", "启动测量", "测量中", "结束"}."结束"] -> w196
                  frame False {
                    n171 = flat-sequence {
                      tunnel: [enum16{"待机", "启动测量", "测量中", "结束"}."测量中"] -> w197
                      frame #0 {
                        n172 = Wait (ms)(milliseconds to wait=u32 1000 ("等待时间（毫秒）")) -> ()  [unwired: 1 out]
                      }
                      frame #1 {
                      }
                    }
                  }
                  frame True {
                  }
                }
              }
              frame "结束" {
                n173 = First Call?() -> (First Call?: T/F=w201:bool)
                n174 = case shown="真" w201 {
                  frame False {
                  }
                  frame True {
                    n175 = Get Date/Time In Seconds() -> (seconds since 1Jan1904=w208:timestamp)
                    n176 = Bundle By Name(cluster=T4 {"时间标识"=timestamp(0 s since 1904-01-01), "设备"="", "日志信息"="", "流程参数"=""} ("data in"), "时间标识"=w208, "设备"="CODCr", "日志信息"="-->>CODCr测量结束") -> (w204:T4)
                    n177 = call "总磷氨氮操作日志.vi"("data in"=w204) -> ()  [unwired: 11 in]
                  }
                }
              }
            }
            n178 = feedback-in #8(w162) -> ()
          }
        }
        n179 = case shown="真" w98 {
          tunnel: w107 -> [_ w211]
          tunnel: [TRUE w210] -> w104
          frame False {
          }
          frame True {
            n180 = feedback #10(T7."待机") -> (w213:T7)
            n181 = case shown="\"氨氮测量中\"" w213 {
              tunnel: [T7."启动氨氮" w226 w261 w300 w335 T7."结束"] -> w212
              tunnel: w211 -> [_ w227 _ w301 _ _]
              tunnel: [_ _ _ _ _ TRUE] -> w210
              frame "待机", Default {
              }
              frame "启动氨氮" {
                n182 = First Call?() -> (First Call?: T/F=w216:bool)
                n183 = case shown="真" w216 {
                  frame False {
                  }
                  frame True {
                    n184 = global read "VAR总磷氨氮全局变量.vi" "总氮状态告警区"() -> (w232:T12)
                    n185 = global read "VAR总磷氨氮全局变量.vi" "总氮测量数据区"() -> (w243:T13)
                    n186 = Unbundle By Name(w232) -> ("id"=w231:u16, "flowid"=w230:u16, "量程"=w229:u16)
                    n187 = Unbundle By Name(w243) -> ("F0"=w241:sgl, "F1"=w240:sgl, "F2"=w239:sgl, "F3"=w238:sgl, "F4"=w237:sgl, "F5"=w236:sgl, "F6"=w235:sgl, "F7"=w234:sgl, "X值"=w233:sgl)
                    n188 = Format Into String(format string="F0=%#f,F1=%#f,F2=%#f,F3=%#f,F4=%#f,F5=%#f,F6=%#f,F7=%#f,X=%#f,Flow=%d-%d-%d" ("格式字符串"), w241, w240, w239, w238, w237, w236, w235, w234, w233, w231, w230, w229) -> (resulting string=w228:string)  [unwired: 2 in, 1 out]
                    n189 = Get Date/Time In Seconds() -> (seconds since 1Jan1904=w246:timestamp)
                    n190 = Bundle By Name(cluster=T4 {"时间标识"=timestamp(0 s since 1904-01-01), "设备"="", "日志信息"="", "流程参数"=""} ("data in"), "时间标识"=w246, "设备"="总氮", "日志信息"="-->>总氮测量开始", "流程参数"=w228) -> (w247:T4)
                    n191 = call "总磷氨氮操作日志.vi"("data in"=w247) -> ()  [unwired: 11 in]
                  }
                }
                n192 = call "总磷氨氮启动命令.vi"("参数"=T8 {"站号"=2, "量程切换"=enum."AUTO", "控制命令"=enum."启动测量", "模式设置"=enum."待机", "测量间隔"=0}) -> ("启动命令"=w217:cluster{"命令":string, "data":variant})  [unwired: 10 in]
                n193 = Enqueue Element(queue=w227, element=w217) -> ()  [unwired: 2 in, 3 out]
                n194 = feedback #11() -> (w223:i32)  [unwired: 1 in]
                n195 = Increment(x=w223) -> (x+1=w222:i32)
                n196 = First Call?() -> (First Call?: T/F=w224:bool)
                n197 = Select(t=0, s=w224, f=w222) -> (s? t:f=w221:i32)
                n198 = feedback-in #11(w221) -> ()
                n199 = Greater Or Equal?(x=w221, y=60) -> (x >= y?=w219:bool)
                n200 = case shown="真" w219 {
                  tunnel: [w251 T7."启动总磷"] -> w226
                  frame False {
                    n201 = global read "VAR总磷氨氮全局变量.vi" "状态告警区"() -> (w254:T12)
                    n202 = Unbundle By Name(w254) -> ("工作状态"=w253:T6)
                    n203 = Not Equal To 0?(x=w253) -> (x != 0?=w252:bool)
                    n204 = Select(t=T7."氨氮测量中", s=w252, f=T7."启动氨氮") -> (s? t:f=w251:T7)
                  }
                  frame True {
                    n205 = Get Date/Time In Seconds() -> (seconds since 1Jan1904=w259:timestamp)
                    n206 = Bundle By Name(cluster=T5 {"时间标识"=timestamp(0 s since 1904-01-01), "设备"="", "日志信息"=""} ("data in"), "时间标识"=w259, "设备"="总氮", "日志信息"="总氮启动失败") -> (w255:T5)
                    n207 = call "总磷氨氮报警信息.vi"("data in"=w255) -> ()  [unwired: 11 in]
                  }
                }
              }
              frame "氨氮测量中" {
                n208 = global read "VAR总磷氨氮全局变量.vi" "状态告警区"() -> (w264:T12)
                n209 = Unbundle By Name(w264) -> ("工作状态"=w263:T6, "id"=w262:u16)
                n210 = case shown="\"空闲\"" w263 {
                  tunnel: [T7."启动总磷" T7."氨氮测量中"] -> w261
                  tunnel: w262 -> [_ _]
                  frame "空闲" {
                    n211 = First Call?() -> (First Call?: T/F=w265:bool)
                    n212 = Wait (ms)(milliseconds to wait=u32 5000 ("等待时间（毫秒）")) -> ()  [unwired: 1 out]
                    n213 = case shown="真" w265 {
                      frame False {
                      }
                      frame True {
                        n214 = global read "VAR总磷氨氮全局变量.vi" "总氮状态告警区"() -> (w272:T12)
                        n215 = global read "VAR总磷氨氮全局变量.vi" "总氮测量数据区"() -> (w283:T13)
                        n216 = Unbundle By Name(w272) -> ("id"=w271:u16, "flowid"=w270:u16, "量程"=w269:u16)
                        n217 = Unbundle By Name(w283) -> ("F0"=w281:sgl, "F1"=w280:sgl, "F2"=w279:sgl, "F3"=w278:sgl, "F4"=w277:sgl, "F5"=w276:sgl, "F6"=w275:sgl, "F7"=w274:sgl, "X值"=w273:sgl)
                        n218 = Format Into String(format string="F0=%#f,F1=%#f,F2=%#f,F3=%#f,F4=%#f,F5=%#f,F6=%#f,F7=%#f,X=%#f,Flow=%d-%d-%d" ("格式字符串"), w281, w280, w279, w278, w277, w276, w275, w274, w273, w271, w270, w269) -> (resulting string=w268:string)  [unwired: 2 in, 1 out]
                        n219 = Get Date/Time In Seconds() -> (seconds since 1Jan1904=w286:timestamp)
                        n220 = Bundle By Name(cluster=T4 {"时间标识"=timestamp(0 s since 1904-01-01), "设备"="", "日志信息"="", "流程参数"=""} ("data in"), "时间标识"=w286, "设备"="总氮", "日志信息"="-->>总氮测量结束", "流程参数"=w268) -> (w287:T4)
                        n221 = call "总磷氨氮操作日志.vi"("data in"=w287) -> ()  [unwired: 11 in]
                      }
                    }
                  }
                  frame "水样测试", Default {
                  }
                }
              }
              frame "启动总磷" {
                n222 = First Call?() -> (First Call?: T/F=w290:bool)
                n223 = case shown="真" w290 {
                  frame False {
                  }
                  frame True {
                    n224 = global read "VAR总磷氨氮全局变量.vi" "总磷状态告警区"() -> (w306:T12)
                    n225 = global read "VAR总磷氨氮全局变量.vi" "总磷测量数据区"() -> (w317:T13)
                    n226 = Unbundle By Name(w306) -> ("id"=w305:u16, "flowid"=w304:u16, "量程"=w303:u16)
                    n227 = Unbundle By Name(w317) -> ("F0"=w315:sgl, "F1"=w314:sgl, "F2"=w313:sgl, "F3"=w312:sgl, "F4"=w311:sgl, "F5"=w310:sgl, "F6"=w309:sgl, "F7"=w308:sgl, "X值"=w307:sgl)
                    n228 = Format Into String(format string="F0=%#f,F1=%#f,F2=%#f,F3=%#f,F4=%#f,F5=%#f,F6=%#f,F7=%#f,X=%#f,Flow=%d-%d-%d" ("格式字符串"), w315, w314, w313, w312, w311, w310, w309, w308, w307, w305, w304, w303) -> (resulting string=w302:string)  [unwired: 2 in, 1 out]
                    n229 = Get Date/Time In Seconds() -> (seconds since 1Jan1904=w320:timestamp)
                    n230 = Bundle By Name(cluster=T4 {"时间标识"=timestamp(0 s since 1904-01-01), "设备"="", "日志信息"="", "流程参数"=""} ("data in"), "时间标识"=w320, "设备"="总磷", "日志信息"="-->>总磷测量开始", "流程参数"=w302) -> (w321:T4)
                    n231 = call "总磷氨氮操作日志.vi"("data in"=w321) -> ()  [unwired: 11 in]
                  }
                }
                n232 = call "总磷氨氮启动命令.vi"("参数"=T8 {"站号"=1, "量程切换"=enum."AUTO", "控制命令"=enum."启动测量", "模式设置"=enum."待机", "测量间隔"=0}) -> ("启动命令"=w291:cluster{"命令":string, "data":variant})  [unwired: 10 in]
                n233 = Enqueue Element(queue=w301, element=w291) -> ()  [unwired: 2 in, 3 out]
                n234 = feedback #12() -> (w297:i32)  [unwired: 1 in]
                n235 = Increment(x=w297) -> (x+1=w296:i32)
                n236 = First Call?() -> (First Call?: T/F=w298:bool)
                n237 = Select(t=0, s=w298, f=w296) -> (s? t:f=w295:i32)
                n238 = feedback-in #12(w295) -> ()
                n239 = Greater Or Equal?(x=w295, y=60) -> (x >= y?=w293:bool)
                n240 = case shown="真" w293 {
                  tunnel: [w325 T7."结束"] -> w300
                  frame False {
                    n241 = global read "VAR总磷氨氮全局变量.vi" "状态告警区"() -> (w326:T12)
                    n242 = Unbundle By Name(w326) -> ("工作状态"=w327:T6)
                    n243 = Not Equal To 0?(x=w327) -> (x != 0?=w328:bool)
                    n244 = Select(t=T7."总磷测量中", s=w328, f=T7."启动总磷") -> (s? t:f=w325:T7)
                  }
                  frame True {
                    n245 = Get Date/Time In Seconds() -> (seconds since 1Jan1904=w334:timestamp)
                    n246 = Bundle By Name(cluster=T5 {"时间标识"=timestamp(0 s since 1904-01-01), "设备"="", "日志信息"=""} ("data in"), "时间标识"=w334, "设备"="总磷", "日志信息"="总磷启动失败") -> (w329:T5)
                    n247 = call "总磷氨氮报警信息.vi"("data in"=w329) -> ()  [unwired: 11 in]
                  }
                }
              }
              frame "总磷测量中" {
                n248 = global read "VAR总磷氨氮全局变量.vi" "状态告警区"() -> (w338:T12)
                n249 = Unbundle By Name(w338) -> ("工作状态"=w337:T6, "id"=w336:u16)
                n250 = case shown="\"水样测试\", 默认" w337 {
                  tunnel: [T7."结束" T7."总磷测量中"] -> w335
                  tunnel: w336 -> [_ _]
                  frame "空闲" {
                  }
                  frame "水样测试", Default {
                  }
                }
              }
              frame "结束" {
                n251 = First Call?() -> (First Call?: T/F=w341:bool)
                n252 = case shown="真" w341 {
                  frame False {
                  }
                  frame True {
                    n253 = global read "VAR总磷氨氮全局变量.vi" "总磷状态告警区"() -> (w348:T12)
                    n254 = global read "VAR总磷氨氮全局变量.vi" "总磷测量数据区"() -> (w359:T13)
                    n255 = Unbundle By Name(w348) -> ("id"=w347:u16, "flowid"=w346:u16, "量程"=w345:u16)
                    n256 = Unbundle By Name(w359) -> ("F0"=w357:sgl, "F1"=w356:sgl, "F2"=w355:sgl, "F3"=w354:sgl, "F4"=w353:sgl, "F5"=w352:sgl, "F6"=w351:sgl, "F7"=w350:sgl, "X值"=w349:sgl)
                    n257 = Format Into String(format string="F0=%#f,F1=%#f,F2=%#f,F3=%#f,F4=%#f,F5=%#f,F6=%#f,F7=%#f,X=%#f,Flow=%d-%d-%d" ("格式字符串"), w357, w356, w355, w354, w353, w352, w351, w350, w349, w347, w346, w345) -> (resulting string=w344:string)  [unwired: 2 in, 1 out]
                    n258 = Get Date/Time In Seconds() -> (seconds since 1Jan1904=w362:timestamp)
                    n259 = Bundle By Name(cluster=T4 {"时间标识"=timestamp(0 s since 1904-01-01), "设备"="", "日志信息"="", "流程参数"=""} ("data in"), "时间标识"=w362, "设备"="总磷", "日志信息"="-->>总磷开始测量", "流程参数"=w344) -> (w363:T4)
                    n260 = call "总磷氨氮操作日志.vi"("data in"=w363) -> ()  [unwired: 11 in]
                  }
                }
              }
            }
            n261 = feedback-in #10(w212) -> ()
          }
        }
        n262 = global read "采配水全局变量.vi" "状态"() -> (w94:T11)
        n263 = Unbundle By Name(w94) -> ("R0"=w93:i16)
        n264 = Equal To 0?(x=w93) -> (x = 0?=w90:bool)
        n265 = Greater?(x=w93, y=i16 6) -> (0:w91:bool)
        n266 = Or(x=w90, y=w91) -> (x .or. y?=w87:bool)
        n267 = Compound Arithmetic op=AND ("复合运算")(w105, w102, w104, w101) -> (w86:bool)
        n268 = And(x=w86, y=w87) -> (x .and. y?=w85:bool)
        n269 = Select(t=enum16{"初始化", "采配水启动", "等待", "配水", "排水", "结束"}."排水" ("枚举"), s=w85, f=w89) -> (s? t:f=w88:enum16{"初始化", "采配水启动", "等待", "配水", "排水", "结束"})
        n270 = Select(t=enum16{"初始化", "采配水启动", "等待", "配水", "排水", "结束"}."结束", s=w109, f=w88) -> (s? t:f=w108:enum16{"初始化", "采配水启动", "等待", "配水", "排水", "结束"})
      }
      frame "排水" {
        n271 = Increment(x=w497) -> (x+1=w493:enum16{"初始化", "采配水启动", "等待", "配水", "排水", "结束"})
        n272 = Enqueue Element At Opposite End(queue=w498, element=T2 {"命令"="单个写入", {"starting address"=302, "holding register value"=1}} ("元素")) -> ()  [unwired: 2 in, 3 out]
        n273 = Select(t=enum16{"初始化", "采配水启动", "等待", "配水", "排水", "结束"}."结束", s=w494, f=w493) -> (s? t:f=w492:enum16{"初始化", "采配水启动", "等待", "配水", "排水", "结束"})
      }
      frame "结束" {
        n274 = case shown="真" w500 {
          tunnel: w501 -> [_ w506]
          frame False {
          }
          frame True {
            n275 = Enqueue Element At Opposite End(queue=w506, element=T2 {"命令"="单个写入", {"starting address"=300, "holding register value"=2}} ("元素")) -> ()  [unwired: 2 in, 3 out]
          }
        }
        n276 = Increment(x=w505) -> (x+1=w504:enum16{"初始化", "采配水启动", "等待", "配水", "排水", "结束"})
      }
    }
    "枚举" <- w31
    n277 = Wait (ms)(milliseconds to wait=u32 1000 ("等待时间（毫秒）")) -> ()  [unwired: 1 out]
    n278 = Format Into String(format string="%s,当前运行时间%d秒" ("格式字符串"), w24, w23) -> (resulting string=w20:string)  [unwired: 2 in, 1 out]
    n279 = global write "采配水全局变量.vi" "运行状态显示"(w20) -> ()
  }
  n280 = Cancel Notification(0:w8) -> (8:w7:refnum<notifier>)  [unwired: 1 in, 2 out]
  n281 = Release Notifier(notifier=w7) -> ()  [unwired: 2 in, 3 out]
